vi "Send stack info.vi"(8 "error in (no error)":errorcluster, 11 "Tomo in":refnum<class "Tomo.lvclass">) -> (0 "error out":errorcluster, 3 "Tomo out":refnum<class "Tomo.lvclass">)   [LabVIEW 2012, in "Tomo.lvclass"]
uses:
  Tomo.lvclass
  <vilib>/Distrio/Murmex/Murmex/update_cluster.ctl
  Tomo.lvclass/Tomo.ctl
  <vilib>/Distrio/Murmex/Murmex/Murmex.lvclass
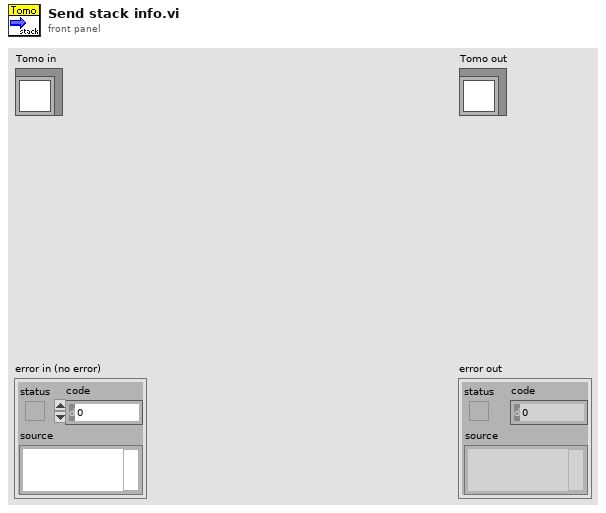
[diagram p1: front panel]
types:
  T1 = typedef "Murmex.lvlib/Murmex.lvclass/update_cluster.ctl" = cluster{"target ID":string, "key chains":string[], "values":variant[]}
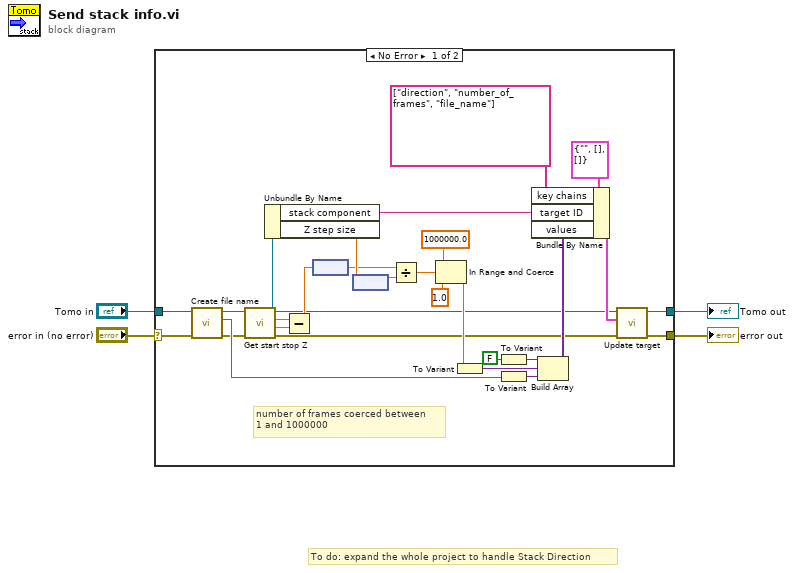
[diagram p0: block diagram]
diagram:
  # "To do: expand the whole project to handle Stack Direction"
  n1 = case shown="No Error" "error in (no error)" {
    selector: "error in (no error)" -> [w6 w34]
    tunnel: [w27 w34] -> w3
    tunnel: [w26 w33] -> w1
    tunnel: "Tomo in" -> [w7 w33]
    frame No Error {
      # "number of frames coerced between\n1 and 1000000"
      n2 = call-dynamic "Create file name.vi"("error in (no error)"=w6, "Tomo in"=w7) -> ("error out"=w14:errorcluster, "filename"=w21:string, "Tomo out"=w12:refnum<class "Tomo.lvclass">)  [unwired: 7 in]
      n3 = call-dynamic "Get start stop Z.vi"("error in (no error)"=w14, "Tomo in"=w12) -> ("error out"=w13:errorcluster, "Z start"=w9:dbl[unit], "Z stop"=w10:dbl[unit], "Tomo out"=w11:refnum<class "Tomo.lvclass">)  [unwired: 4 in, 2 out]
      n4 = Unbundle By Name(w11) -> ("stack component"=w24:string, "Z step size"=w32:dbl[unit])
      n5 = Subtract(x=w10, y=w9) -> (x-y=w18:dbl[unit])
      n6 = node(w18) -> (w8:dbl)
      n7 = node(w32) -> (w19:dbl)
      n8 = Divide(x=w8, y=w19) -> (x/y=w5:dbl)
      n9 = In Range and Coerce(upper limit=1000000.0, x=w5, lower limit=1.0) -> (coerced(x)=w17:dbl)  [unwired: 1 out]
      n10 = To Variant(anything=w17) -> (Variant=w30:variant)
      n11 = To Variant(anything=FALSE ("x = 0?")) -> (Variant=w23:variant)
      n12 = To Variant(anything=w21) -> (Variant=w22:variant)
      n13 = Build Array(w23, w30, w22) -> (w29:variant[])
      n14 = Bundle By Name(cluster=T1 {"target ID"="", "key chains"=[], "values"=[]} ("update cluster"), "key chains"=string[] ["direction", "number_of_frames", "file_name"], "target ID"=w24, "values"=w29) -> (w31:T1)
      n15 = call <vilib>:"Update target.vi"("error in (no error)"=w13, "update cluster"=w31, "MurmexBase in"=w11) -> ("error out"=w27:errorcluster, "MurmexBase out"=w26:refnum<class "Tomo.lvclass">)  [unwired: 7 in]
    }
    frame Error {
    }
  }
  "error out" <- w3
  "Tomo out" <- w1
